vi "Print Switch Finished.vi"(8 "error in (no error)":errorcluster, 10 "State":bool, 11 "Main.lvlib:Main.lvclass":refnum<class "Main.lvclass">) -> (0 "error out":errorcluster, 3 "Main.lvlib:Main.lvclass 2":refnum<class "Main.lvclass">)   [LabVIEW 2018, in "Main.lvlib" / "Main.lvclass"]
uses:
  Main.lvclass
  Main.lvclass/Main.ctl
  Stage Actor/Stage Messages/Set Digital Inputs Msg/Set Digital Inputs Msg.lvclass
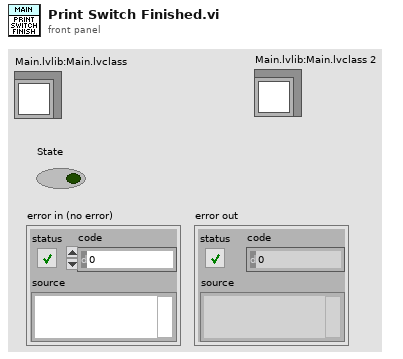
[diagram p1: front panel]
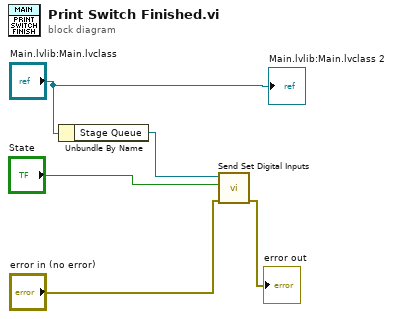
[diagram p0: block diagram]
diagram:
  n1 = Unbundle By Name("Main.lvlib:Main.lvclass") -> ("Stage Queue"=w5:refnum<class "Message Enqueuer.lvclass">)
  n2 = call "Send Set Digital Inputs.vi"("error in (no error)"="error in (no error)", "State"="State", "Message Enqueuer in"=w5) -> ("error out"=→"error out":errorcluster)  [unwired: 7 in, 1 out]
  "Main.lvlib:Main.lvclass 2" <- "Main.lvlib:Main.lvclass"
